vi "peaks_and_crossings.vi"(7 "width":i32=3 min=3, 8 "crossing level":dbl, 9 "end":dbl=1.0, 10 "threshold":dbl=0.25 format="%0.2f", 11 "waveform":waveform(dbl)={"t0"=timestamp(3680839669.4856114 s since 1904-01-01), "dt"=0.009575387048624538, "Y"=array[27346 elements]}) -> (0 "crossings":dbl[](array[numeric]), 1 "mean of peaks":dbl format="%0.2f", 2 "all in array":cluster{dbl[], "Amplitudes":dbl[]}[](array[cluster]), 3 "peak locations":dbl[](array[numeric]), 4 "plus-minus crossing?":bool[](array[boolean]), 5 "standard deviation of peaks":dbl format="%0.2f", 6 "minus-plus crossing?":bool[](array[boolean]))   [LabVIEW 2020]
uses:
  <vilib>/Analysis/1siggen.llb/Ramp Pattern by Delta.vi
  <vilib>/Analysis/NI_AAL_SigProc.lvlib
  <vilib>/Analysis/NI_AALBase.lvlib
panel:
  out "inspection":cluster{"Y":dbl[], "Y":dbl[]}[](graph)
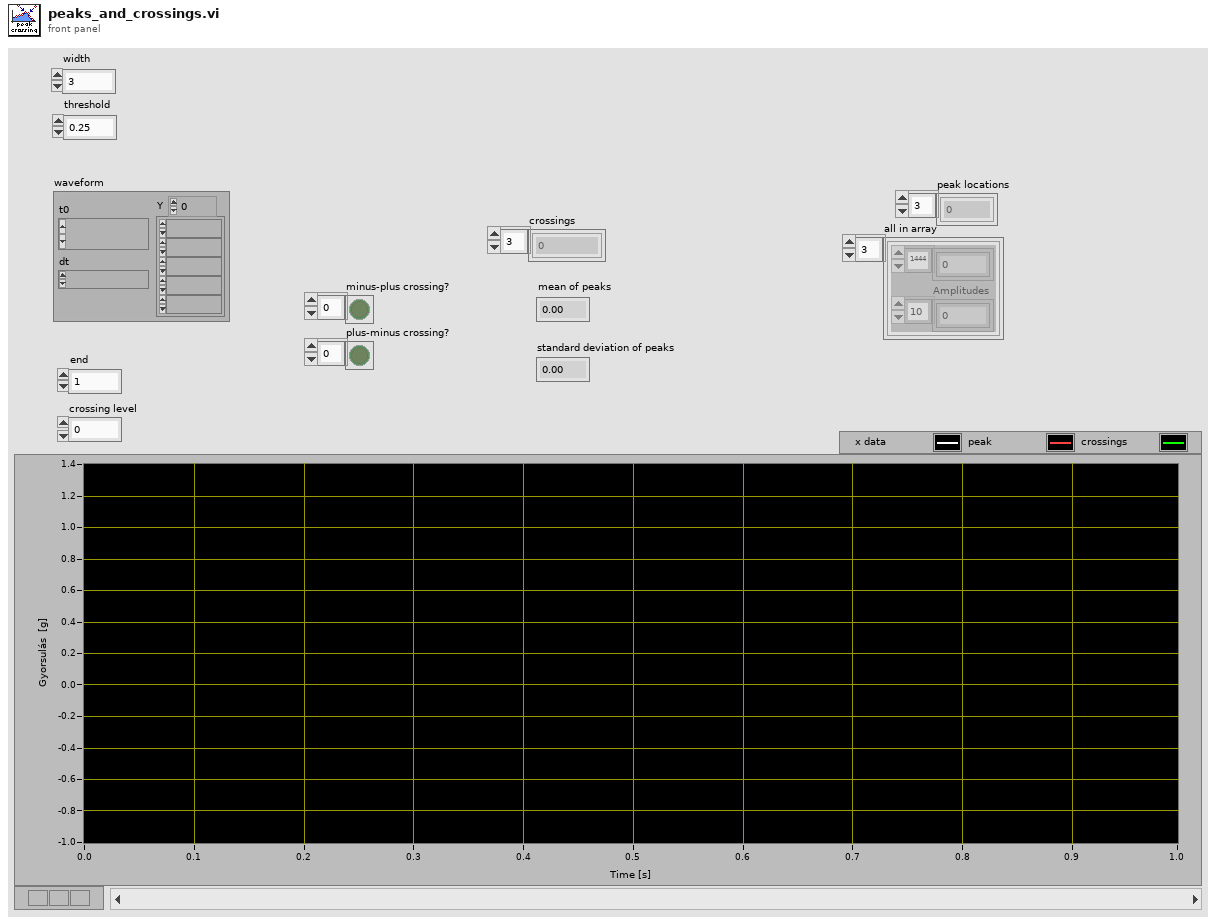
[diagram p1: front panel]
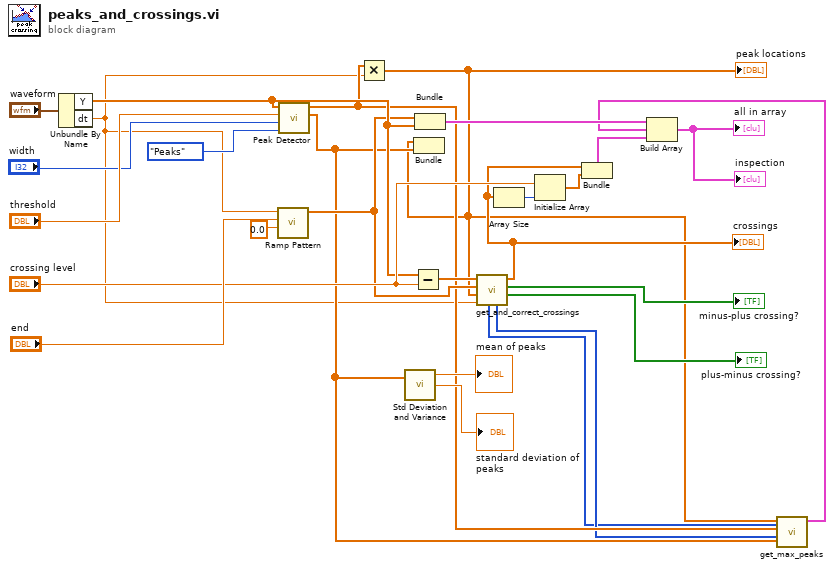
[diagram p0: block diagram]
diagram:
  n1 = Unbundle By Name("waveform") -> ("Y"=w16:dbl[], "dt"=w4:dbl)
  n2 = call-poly <vilib>:"Ramp Pattern.vi"("start"=0.0, "end"="end", "delta"=w4) -> ("Ramp Pattern"=w12:dbl[])  [unwired: 6 in, 2 out]
  n3 = call <vilib>:"Peak Detector.vi"("peaks/valleys"=enum32{"Peaks", "Valleys"}."Peaks", "width"="width", "threshold"="threshold", "X"=w16) -> ("Amplitudes"=w8:dbl[], "Locations"=w6:dbl[])  [unwired: 3 in, 3 out]
  n4 = Multiply(x=w6, y=w4) -> (x*y=w5:dbl[])
  "peak locations" <- w5
  n5 = call <vilib>:"Std Deviation and Variance.vi"("X"=w8) -> ("mean"=→"mean of peaks":dbl, "standard deviation"=→"standard deviation of peaks":dbl)  [unwired: 1 in, 1 out]
  n6 = Subtract(x=w16, y="crossing level") -> (x-y=w13:dbl[])
  n7 = Bundle(w5, "Amplitudes"=w8) -> ()  [unwired: 1 in, 1 out]
  n8 = Bundle("Ramp Pattern"=w12, "Y"=w16) -> (w7:cluster{"Ramp Pattern":dbl[], "Y":dbl[]})  [unwired: 1 in]
  n9 = call "get_and_correct_crossings.vi"("dt"=w4, "peak times"=w5, "signal index"=w12, "singal"=w13) -> ("p->n crossing?"=→"plus-minus crossing?":bool[], "n->p crossing?"=→"minus-plus crossing?":bool[], "crossings"=w11:dbl[], "p->n indexes"=w3:i32[], "n->p indexes"=w2:i32[])  [unwired: 3 in]
  "crossings" <- w11
  n10 = Array Size(array=w11) -> (size(s)=w19:i32)
  n11 = Initialize Array("crossing level", w19) -> (w21:dbl[])
  n12 = Bundle("crossings"=w11, w21) -> (w22:cluster{"crossings":dbl[], dbl[]})  [unwired: 1 in]
  n13 = call "get_max_peaks.vi"("Amplitudes"=w8, "n->p indexes"=w2, "p->n indexes"=w3, "Locations"=w6, "peak times"=w5) -> ("Correted Peaks"=w1:cluster{"Array":dbl[], "Array":dbl[]})  [unwired: 5 in, 1 out]
  n14 = Build Array(w7, w1, w22) -> (→"all in array" →"inspection":cluster{"crossings":dbl[], "Array":dbl[]}[])
